vi "ListSetTimebase.vi"(3 "error in (no error)":errorcluster, 4 "Timebase":enum16{"Time", "Cycles"}(ring), 5 "VISA resource name":refnum<visa-resource-name>) -> (0 "error out":errorcluster, 2 "VISA resource name out":refnum<visa-resource-name>)   [LabVIEW 2018, in "BK Precision 983X Series.lvlib"]
uses:
  <instrlib>/BK Precision 983X Series/BK Precision 983X Series.lvlib
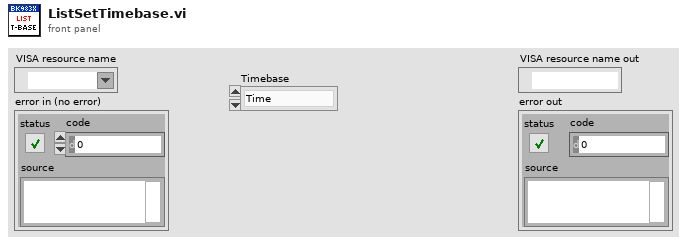
[diagram p1: front panel]
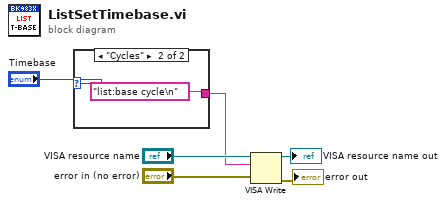
[diagram p0: block diagram]
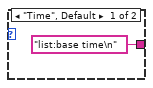
[diagram p2: hidden frame]
diagram:
  n1 = case shown="\"Cycles\"" "Timebase" {
    tunnel: ["list:base time\n" ("write buffer") "list:base cycle\n" ("write buffer")] -> w1
    frame "Time", Default {
    }
    frame "Cycles" {
    }
  }
  n2 = VISA Write(VISA resource name="VISA resource name", write buffer=w1, error in (no error)="error in (no error)") -> (VISA resource name out=→"VISA resource name out":refnum<visa-resource-name>, error out=→"error out":errorcluster)  [unwired: 1 out]
